vi "Send-heartbeat.vi"(8 "error in (no error)":errorcluster, 11 "Client in":T1) -> (0 "error out":errorcluster, 3 "Client out":T1)   [LabVIEW 2013, in "SLMControl.lvlib" / "SC-Client.lvclass"]
doc: "Wrapper function for sending the specific 'Hearbeat' type message.\nThis function creates and immediately sends a heartbeat message to the server, using the configuration of the client object."
uses:
  SC-Client.lvclass
  Object-reference.ctl
  SC-Client.lvclass/SC-Client.ctl
  SA-SLMAPI/Sources/Heartbeat/Heartbeat.lvclass
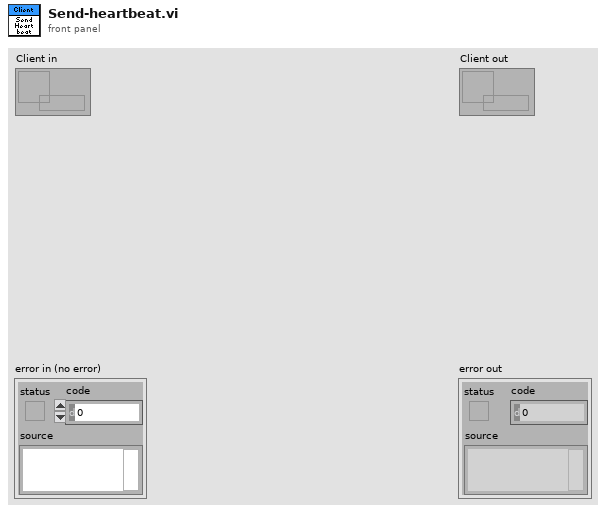
[diagram p1: front panel]
types:
  T1 = typedef "SLMControl.lvlib/SC-Client.lvclass/Object-reference.ctl" = refnum<data-value>
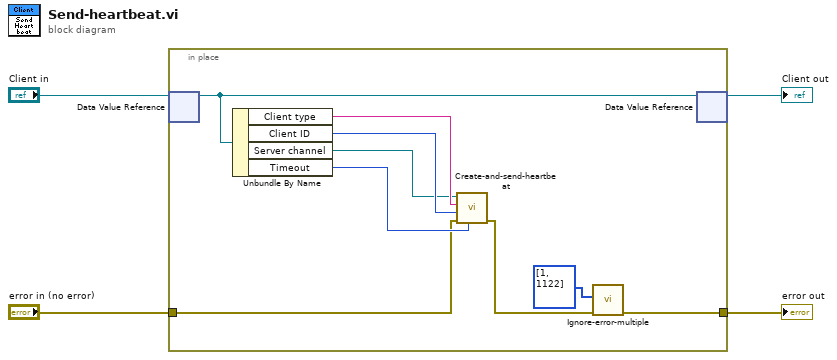
[diagram p0: block diagram]
diagram:
  n1 = in-place {
    in-place-border: "error in (no error)" -> [w9]
    in-place-border: [w6] -> w3
    n2 = in-place-dvr #1("Client in") -> (w7:refnum<class "SC-Client.lvclass">)  [unwired: 1 out]
    n3 = Unbundle By Name(w7) -> ("Client type"=w13:string, "Client ID"=w12:i32, "Server channel"=w11:refnum<queue>, "Timeout"=w10:i32)
    n4 = call "Create-and-send-heartbeat.vi"("Timeout"=w10, "error in (no error)"=w9, "Sender ID"=w12, "Sender"=w13, "Server channel"=w11) -> ("error out"=w8:errorcluster)  [unwired: 6 in]
    n5 = call "Ignore-error-multiple.vi"("error in (no error)"=w8, "Errors to ignore (1)"=i32[] [1, 1122]) -> ("error out"=w6:errorcluster)  [unwired: 9 in]
    n6 = in-place-dvr #1(w7) -> (→"Client out":T1)  [unwired: 1 out]
  }
  "error out" <- w3
